vi "Read Active Project.vi"(11 "Project Stuff in":refnum<class "Project Stuff.lvclass">) -> (2 "Active Project":refnum<vi>)   [LabVIEW 2025, in "_Shared.lvlib" / "Project Stuff.lvclass"]
uses:
  Project Stuff.lvclass
  Project Stuff.lvclass/Project Stuff.ctl
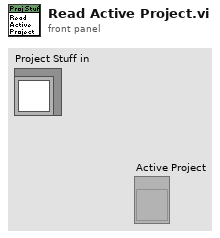
[diagram p1: front panel]
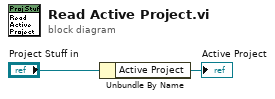
[diagram p0: block diagram]
diagram:
  n1 = Unbundle By Name("Project Stuff in") -> ("Active Project"=→"Active Project":refnum<vi>)
